vi "Update Parameters XML Parsing Error.vi"(8 "error in":errorcluster, 10 "Ports":T1[](array[typedef]) {"Labels"."Label (octal)" format="%o"}, 11 "Configuration files Ref":T5 format="%.0x") -> (0 "error out":errorcluster, 2 "XML error?":bool, 3 "Configuration files Ref out":T5 format="%.0x")   [LabVIEW 2020, in "Ballard ARINC 429 System Explorer.lvlib" / "Implementation.lvlib"]
uses:
  Implementation.lvlib
  <vilib>/NI VeriStand/Custom Device API/Custom Device Item Ref.ctl
  Types/XML Port.ctl
  Types/XML Label.ctl
  Types/XML Parameter.ctl
  Encoding and Decoding/Encoding.ctl
  c0d2c730-0f3c-4a8a-bc57-43fc65a05588.vi
  <vilib>/NI VeriStand/Custom Device API/Custom Device API.lvlib
  Encoding and Decoding/Encoding and Decoding.lvlib
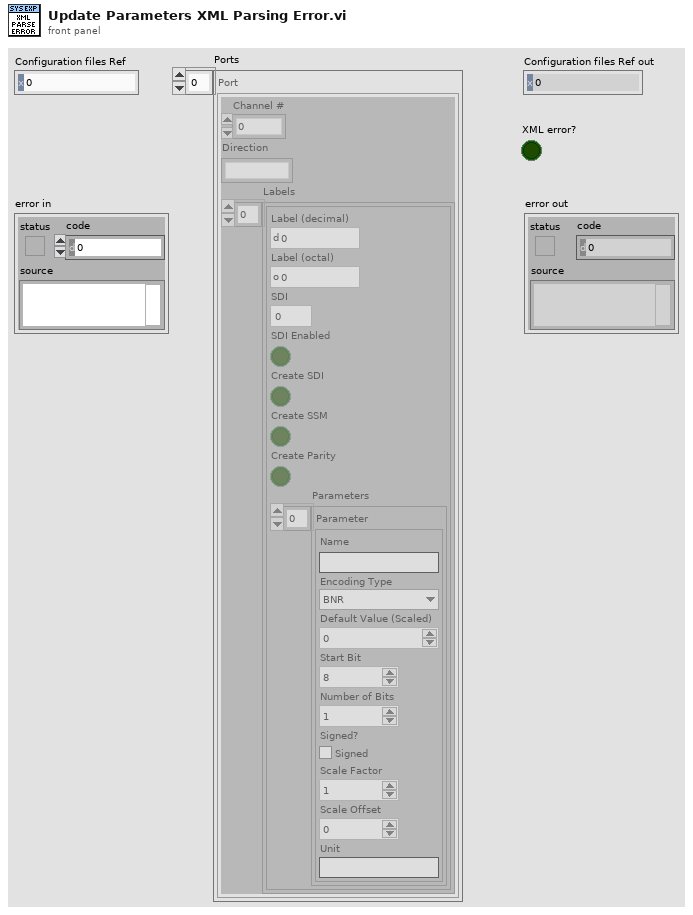
[diagram p1: front panel]
types:
  T1 = typedef "Ballard ARINC 429 System Explorer.lvlib/Implementation.lvlib/XML Port.ctl" = cluster{"Channel #":u16, "Direction":string, "Labels":T2[]}
  T2 = typedef "Ballard ARINC 429 System Explorer.lvlib/Implementation.lvlib/XML Label.ctl" = cluster{"Label (decimal)":i32, "Label (octal)":i32, "SDI":u8, "SDI Enabled":bool, "Create SDI":bool, "Create SSM":bool, "Create Parity":bool, "Parameters":T3[]}
  T3 = typedef "Ballard ARINC 429 System Explorer.lvlib/Implementation.lvlib/XML Parameter.ctl" = cluster{"Name":string, "Encoding Type":T4, "Default Value (Scaled)":dbl, "Start Bit":i32, "Number of Bits":i32, "Signed?":bool, "Scale Factor":dbl, "Scale Offset":dbl, "Unit":string}
  T4 = typedef "Encoding and Decoding.lvlib/Encoding.ctl" = enum16{"BNR", "BCD", "Discrete"}
  T5 = typedef "Custom Device API.lvlib/Custom Device Item Ref.ctl" = u64
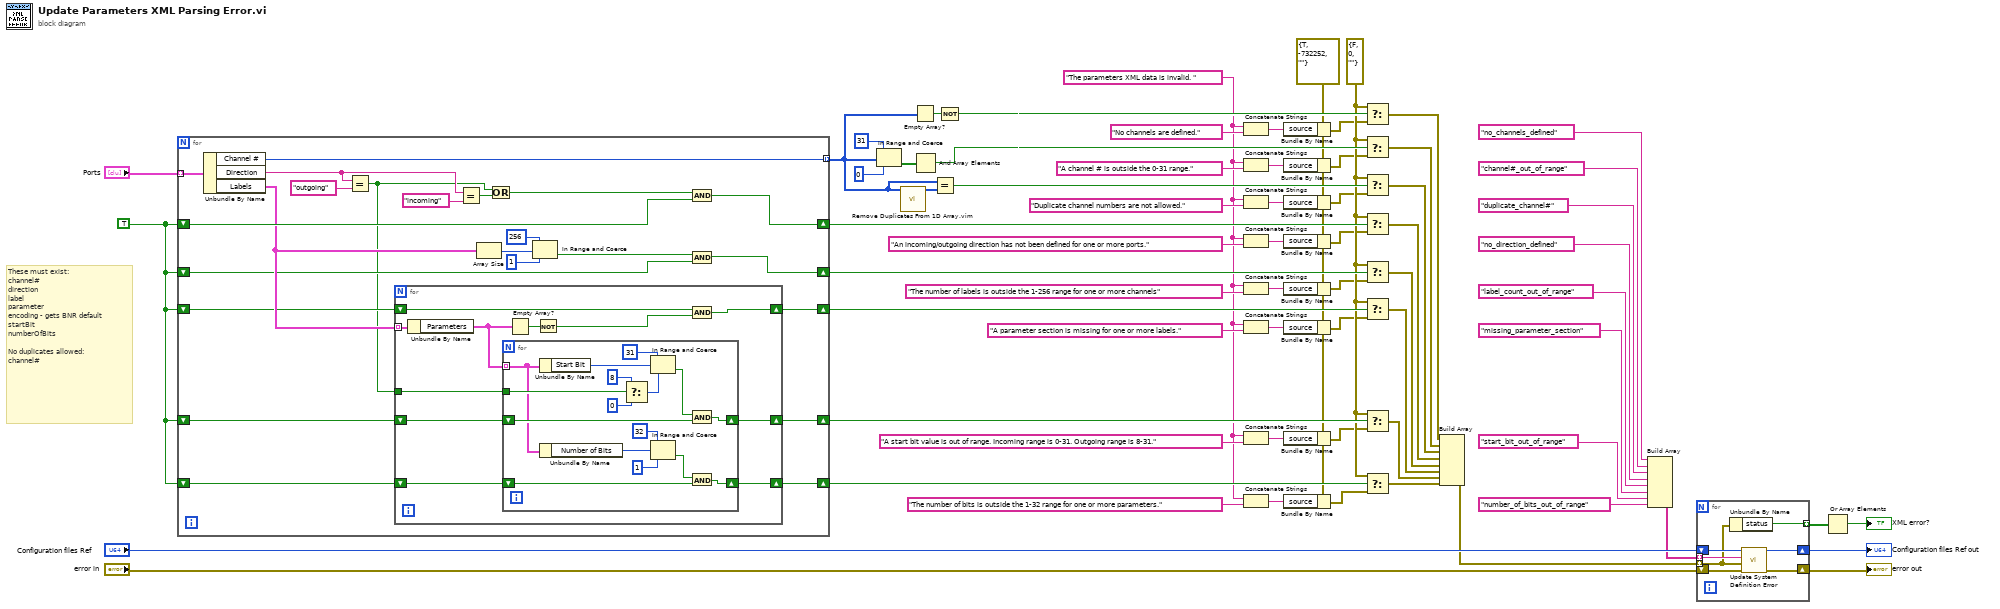
[diagram p0: block diagram]
diagram:
  w22 = errorcluster {"status"=TRUE, "code"=-732252, "source"=""} ("error constant")
  w47 = errorcluster {"status"=FALSE, "code"=0, "source"=""} ("error constant")
  w49 = TRUE
  w21 = "The parameters XML data is invalid. " ("source")
  # "These must exist:\nchannel#\ndirection\nlabel\nparameter\nencoding - gets BNR default\nstartBit\nnumberOfBits\n\nNo duplicates allowed:\nchannel#"
  n1 = for {
    tunnel: "Ports" -> [w90] mode=indexing
    tunnel: [w89] -> w55 mode=indexing
    shift-right: [w84] -> w57
    shift-left: w49 -> [w83]
    shift-right: [w75] -> w52
    shift-left: w49 -> [w76]
    shift-right: [w73] -> w51
    shift-left: w49 -> [w74]
    shift-right: [w70] -> w50
    shift-left: w49 -> [w71]
    shift-right: [w68] -> w48
    shift-left: w49 -> [w69]
    n2 = Unbundle By Name(w90) -> ("Channel #"=w89:u16, "Direction"=w82:string, "Labels"=w81:T2[])
    n3 = Equal?(x=w82, y="outgoing") -> (x = y?=w72:bool)
    n4 = for {
      tunnel: w81 -> [w101] mode=indexing
      shift-right: [w96] -> w73
      shift-left: w74 -> [w97]
      tunnel: w72 -> [w95]
      shift-right: [w93] -> w70
      shift-left: w71 -> [w94]
      shift-right: [w91] -> w68
      shift-left: w69 -> [w92]
      n5 = Unbundle By Name(w101) -> ("Parameters"=w100:T3[])
      n6 = for {
        tunnel: w100 -> [w108] mode=indexing
        tunnel: w95 -> [w116]
        shift-right: [w109] -> w93
        shift-left: w94 -> [w111]
        shift-right: [w102] -> w91
        shift-left: w92 -> [w103]
        n7 = Unbundle By Name(w108) -> ("Start Bit"=w117:i32)
        n8 = Unbundle By Name(w108) -> ("Number of Bits"=w107:i32)
        n9 = Select(t=8 ("Channel #"), s=w116, f=0 ("Channel #")) -> (s? t:f=w112:i32)
        n10 = In Range and Coerce(upper limit=31 ("Channel #"), x=w117, lower limit=w112) -> (In Range?=w110:bool)  [unwired: 1 out]
        n11 = In Range and Coerce(upper limit=32 ("lower limit"), x=w107, lower limit=1) -> (In Range?=w104:bool)  [unwired: 1 out]
        n12 = And(x=w110, y=w111) -> (x .and. y?=w109:bool)
        n13 = And(x=w104, y=w103) -> (x .and. y?=w102:bool)
      }
      n14 = Empty Array?(array=w100) -> (empty?=w99:bool)
      n15 = Not(x=w99) -> (.not. x?=w98:bool)
      n16 = And(x=w97, y=w98) -> (x .and. y?=w96:bool)
    }
    n17 = Equal?(x=w82, y="incoming") -> (x = y?=w88:bool)
    n18 = Array Size(array=w81) -> (size(s)=w80:i32)
    n19 = Or(x=w72, y=w88) -> (x .or. y?=w85:bool)
    n20 = In Range and Coerce(upper limit=256 ("Channel #"), x=w80, lower limit=1 ("Channel #")) -> (In Range?=w77:bool)  [unwired: 1 out]
    n21 = And(x=w85, y=w83) -> (x .and. y?=w84:bool)
    n22 = And(x=w77, y=w76) -> (x .and. y?=w75:bool)
  }
  n23 = In Range and Coerce(upper limit=31 ("Channel #"), x=w55, lower limit=0 ("Channel #")) -> (In Range?=w59:bool[])  [unwired: 1 out]
  n24 = call "Remove Duplicates From 1D Array.vim"("array"=w55) -> ("array with duplicates removed"=w61:u16[])  [unwired: 10 in]
  n25 = Empty Array?(array=w55) -> (empty?=w54:bool)
  n26 = And Array Elements(Boolean array=w59) -> (logical AND=w58:bool)
  n27 = Equal?(x=w55, y=w61) -> (x = y?=w60:bool)
  n28 = Not(x=w54) -> (.not. x?=w53:bool)
  n29 = Concatenate Strings(w21, "No channels are defined." ("source")) -> (w46:string)
  n30 = Concatenate Strings(w21, "A channel # is outside the 0-31 range." ("source")) -> (w43:string)
  n31 = Concatenate Strings(w21, "Duplicate channel numbers are not allowed." ("source")) -> (w41:string)
  n32 = Concatenate Strings(w21, "An incoming/outgoing direction has not been defined for one or more ports." ("source")) -> (w36:string)
  n33 = Concatenate Strings(w21, "The number of labels is outside the 1-256 range for one or more channels" ("source")) -> (w34:string)
  n34 = Concatenate Strings(w21, "A parameter section is missing for one or more labels." ("source")) -> (w30:string)
  n35 = Concatenate Strings(w21, "A start bit value is out of range. Incoming range is 0-31. Outgoing range is 8-31." ("source")) -> (w28:string)
  n36 = Concatenate Strings(w21, "The number of bits is outside the 1-32 range for one or more parameters." ("source")) -> (w24:string)
  n37 = Bundle By Name(cluster=w22, "source"=w46) -> (w42:errorcluster)
  n38 = Bundle By Name(cluster=w22, "source"=w43) -> (w39:errorcluster)
  n39 = Bundle By Name(cluster=w22, "source"=w41) -> (w38:errorcluster)
  n40 = Bundle By Name(cluster=w22, "source"=w36) -> (w35:errorcluster)
  n41 = Bundle By Name(cluster=w22, "source"=w34) -> (w32:errorcluster)
  n42 = Bundle By Name(cluster=w22, "source"=w30) -> (w29:errorcluster)
  n43 = Bundle By Name(cluster=w22, "source"=w28) -> (w26:errorcluster)
  n44 = Bundle By Name(cluster=w22, "source"=w24) -> (w23:errorcluster)
  n45 = Select(t=w47, s=w53, f=w42) -> (s? t:f=w13:errorcluster)
  n46 = Select(t=w47, s=w58, f=w39) -> (s? t:f=w14:errorcluster)
  n47 = Select(t=w47, s=w60, f=w38) -> (s? t:f=w15:errorcluster)
  n48 = Select(t=w47, s=w57, f=w35) -> (s? t:f=w16:errorcluster)
  n49 = Select(t=w47, s=w52, f=w32) -> (s? t:f=w5:errorcluster)
  n50 = Select(t=w47, s=w51, f=w29) -> (s? t:f=w17:errorcluster)
  n51 = Select(t=w47, s=w50, f=w26) -> (s? t:f=w18:errorcluster)
  n52 = Select(t=w47, s=w48, f=w23) -> (s? t:f=w19:errorcluster)
  n53 = Build Array(w13, w14, w15, w16, w5, w17, w18, w19) -> (w4:errorcluster[])
  n54 = Build Array("no_channels_defined" ("error key"), "channel#_out_of_range" ("error key"), "duplicate_channel#" ("error key"), "no_direction_defined" ("error key"), "label_count_out_of_range" ("error key"), "missing_parameter_section" ("error key"), "start_bit_out_of_range" ("error key"), "number_of_bits_out_of_range" ("error key")) -> (w3:string[])
  n55 = for {
    shift-right: [w122] -> w65
    shift-left: "error in" -> [w124]
    shift-right: [w123] -> w66
    shift-left: "Configuration files Ref" -> [w121]
    tunnel: w4 -> [w119] mode=indexing
    tunnel: w3 -> [w120] mode=indexing
    tunnel: [w118] -> w2 mode=indexing
    n56 = Unbundle By Name(w119) -> ("status"=w118:bool)
    n57 = call "Update System Definition Error.vi"("error to report"=w124, "error in"=w119, "error key"=w120, "Configuration files Ref"=w121) -> ("error out"=w122:errorcluster, "Configuration files Ref out"=w123:T5)  [unwired: 6 in]
  }
  "error out" <- w65
  "Configuration files Ref out" <- w66
  n58 = Or Array Elements(Boolean array=w2) -> (logical OR=→"XML error?":bool)
